vi "Cfg List _ Click Symbol.vi"(8 "错误输入":errorcluster caption="错误输入（无错误）", 10 "坐标":T2, 11 "TreeRef":refnum<vi>) -> (0 "错误输出":errorcluster, 1 "Cluster":T1, 2 "Click Colum":string)   [LabVIEW 2016]
uses:
  <vilib>/Utility/miscctls.llb/LVPoint32TypeDef.ctl
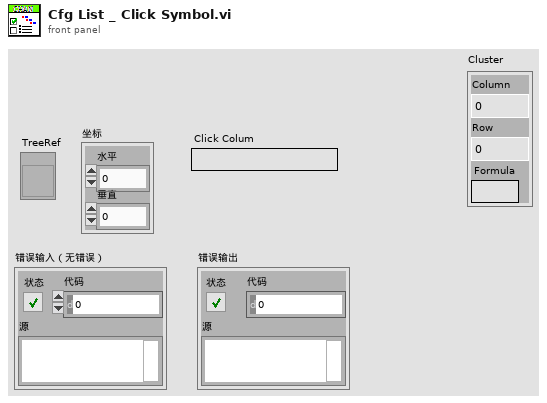
[diagram p1: front panel]
types:
  T1 = cluster{"Column":i32, "Row":i32, "Formula":string}
  T2 = typedef "LVPoint32TypeDef.ctl" = cluster{"Horizontal":i32, "Vertical":i32}
  T3 = cluster{"Col":i32, "Active Item Row Number":i32, "Cell String":string}
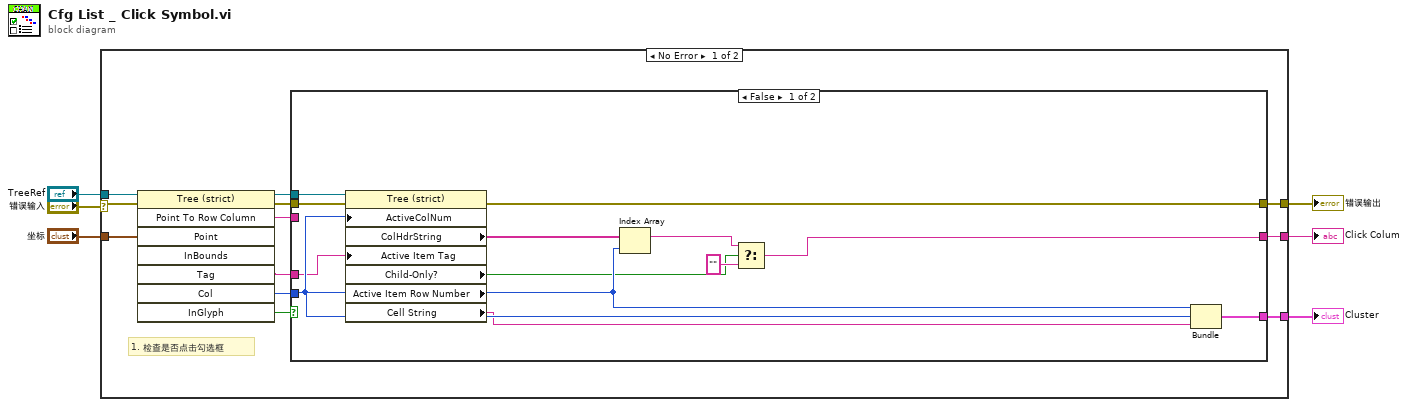
[diagram p0: block diagram]
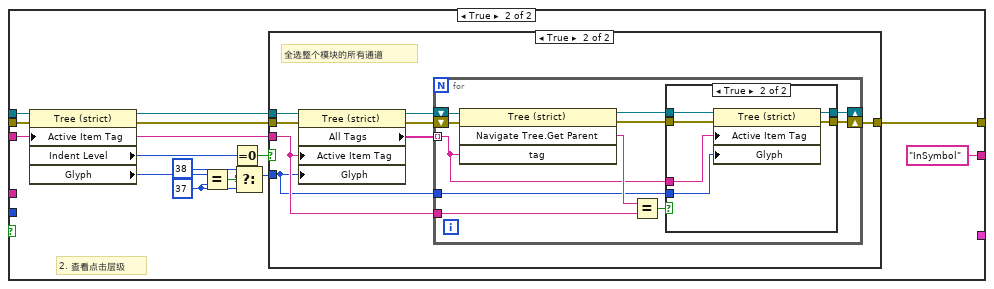
[diagram p2: hidden frame]
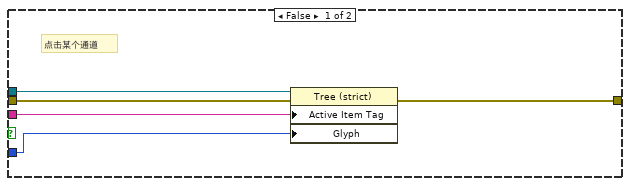
[diagram p3: hidden frame]
diagram:
  n1 = case shown="No Error" "错误输入" {
    selector: "错误输入" -> [w13 w77]
    tunnel: "TreeRef" -> [w17 _]
    tunnel: [w16 w77] -> w5
    tunnel: "坐标" -> [w14 _]
    tunnel: [w9 _] -> w2
    tunnel: [w8 _] -> w1
    frame No Error {
      # "1. 检查是否点击勾选框"
      n2 = invoke class="Tree (strict)" method="Point To Row Column"(reference=w17, error in=w13, "Point"=w14) -> (reference out=w15:refnum<vi>, error out=w12:errorcluster, "Tag"=w7:string, "Col"=w10:i32, "InGlyph"=w11:bool)  [unwired: 5 in, 3 out]
      n3 = case shown="False" w11 {
        tunnel: [w28 w32] -> w16
        tunnel: w15 -> [w30 w44]
        tunnel: w7 -> [_ w33]
        tunnel: w12 -> [w29 w43]
        tunnel: w10 -> [w26 _]
        tunnel: [w19 "InSymbol" ("Cell String")] -> w9
        tunnel: [w23 _] -> w8
        tunnel: w7 -> [w22 _]
        frame False {
          n4 = property class="Tree (strict)"(reference=w30, error in=w29, "ActiveColNum"=w26, "Active Item Tag"=w22) -> (error out=w28:errorcluster, "ColHdrString"=w27:string[], "Child-Only?"=w18:bool, "Active Item Row Number"=w25:i32, "Cell String"=w24:string)  [unwired: 1 out]
          n5 = Index Array(array=w27, index=w26) -> (element=w20:string)
          n6 = Select(t=w20, s=w18, f="") -> (s? t:f=w19:string)
          n7 = Bundle("Col"=w26, "Active Item Row Number"=w25, "Cell String"=w24) -> (w23:T3)  [unwired: 1 in]
        }
        frame True {
          w35 = 37 ("y")
          # "2. 查看点击层级"
          n8 = property class="Tree (strict)"(reference=w44, error in=w43, "Active Item Tag"=w33) -> (reference out=w40:refnum<vi>, error out=w39:errorcluster, "Indent Level"=w42:i32, "Glyph"=w38:i32)
          n9 = Equal?(x=w38, y=w35) -> (x = y?=w37:bool)
          n10 = Equal To 0?(x=w42) -> (x = 0?=w41:bool)
          n11 = Select(t=38 ("y"), s=w37, f=w35) -> (s? t:f=w34:i32)
          n12 = case shown="True" w41 {
            tunnel: w40 -> [w49 w57]
            tunnel: w39 -> [w48 w56]
            tunnel: w34 -> [w47 w51]
            tunnel: w33 -> [w46 w52]
            tunnel: [w45 w50] -> w32
            frame False {
              # "点击某个通道"
              n13 = property class="Tree (strict)"(reference=w49, error in=w48, "Active Item Tag"=w46, "Glyph"=w47) -> (error out=w45:errorcluster)  [unwired: 1 out]
            }
            frame True {
              # "全选整个模块的所有通道"
              n14 = property class="Tree (strict)"(reference=w57, error in=w56, "Active Item Tag"=w52, "Glyph"=w51) -> (reference out=w55:refnum<vi>, error out=w54:errorcluster, "All Tags"=w53:string[])
              n15 = for {
                shift-right: [w62] -> _
                shift-left: w55 -> [w68]
                tunnel: w53 -> [w59] mode=indexing
                tunnel: w52 -> [w65]
                shift-right: [w61] -> w50
                shift-left: w54 -> [w67]
                tunnel: w51 -> [w58]
                n16 = invoke class="Tree (strict)" method="Navigate Tree.Get Parent"(reference=w68, error in=w67, "tag"=w59) -> (reference out=w64:refnum<vi>, error out=w63:errorcluster, "Navigate Tree:Get Parent"=w66:string)  [unwired: 1 in, 1 out]
                n17 = Equal?(x=w66, y=w65) -> (x = y?=w60:bool)
                n18 = case shown="True" w60 {
                  tunnel: w64 -> [w70 w76]
                  tunnel: w63 -> [w69 w75]
                  tunnel: [w70 w74] -> w62
                  tunnel: [w69 w73] -> w61
                  tunnel: w59 -> [_ w72]
                  tunnel: w58 -> [_ w71]
                  frame False {
                  }
                  frame True {
                    n19 = property class="Tree (strict)"(reference=w76, error in=w75, "Active Item Tag"=w72, "Glyph"=w71) -> (reference out=w74:refnum<vi>, error out=w73:errorcluster)
                  }
                }
              }
            }
          }
        }
      }
    }
    frame Error {
    }
  }
  "错误输出" <- w5
  "Click Colum" <- w2
  "Cluster" <- w1
